vi "KB-CalArrayPointXY.vi"(6 "子数组":dbl[][](array[numeric]), 8 "error in (no error)":errorcluster caption="错误输入（无错误）", 9 "Point":cluster{"X":dbl, "Y":dbl, "Z":dbl}[](array[cluster]), 11 "Image In":T1(plugin-control)) -> (0 "error out":errorcluster caption="错误输出", 1 "Z1-Z2":dbl, 2 "H":string, 3 "Image Out":T1(plugin-control), 4 "对角面最高点":cluster{"X":dbl, "Y":dbl, "Z":dbl})   [LabVIEW 2015]
uses:
  <vilib>/Math Plots/3D Math Plots/3D Surface/3D Surface XCtrl/3D Surface.xctl
  <vilib>/Math Plots/3D Math Plots/3D Surface/3D Surface Datatype/Public/Plot Helper (Matrix).vi
  <vilib>/Math Plots/3D Math Plots/3D Surface/3D Surface Datatype/3D Surface Datatype.lvclass
panel:
  out "子数组 3":dbl[][](array[numeric])
  out "3D Surface 3":refnum<class "3D Plot Datatype.lvclass">[](xcontrol) caption="三维曲面"
  out "最大值":dbl
  out "最大索引":i32[](array[numeric])
  out "3D Surface 2":refnum<class "3D Plot Datatype.lvclass">[](xcontrol) caption="三维曲面"
  out "3D Surface":refnum<class "3D Plot Datatype.lvclass">[](xcontrol) caption="三维曲面"
  out "元素 3":dbl
  out "子数组 2":dbl[][](array[numeric])
  out "x与y？ 4":bool
  out "x与y？ 3":bool
  out "x与y？ 2":bool
  out "x与y？":bool
  out "数字":u32
  out "2R":i32
  out "大小":i32[](array[numeric])
  out "最高点":cluster{"X":dbl, "Y":dbl, "Z":dbl}
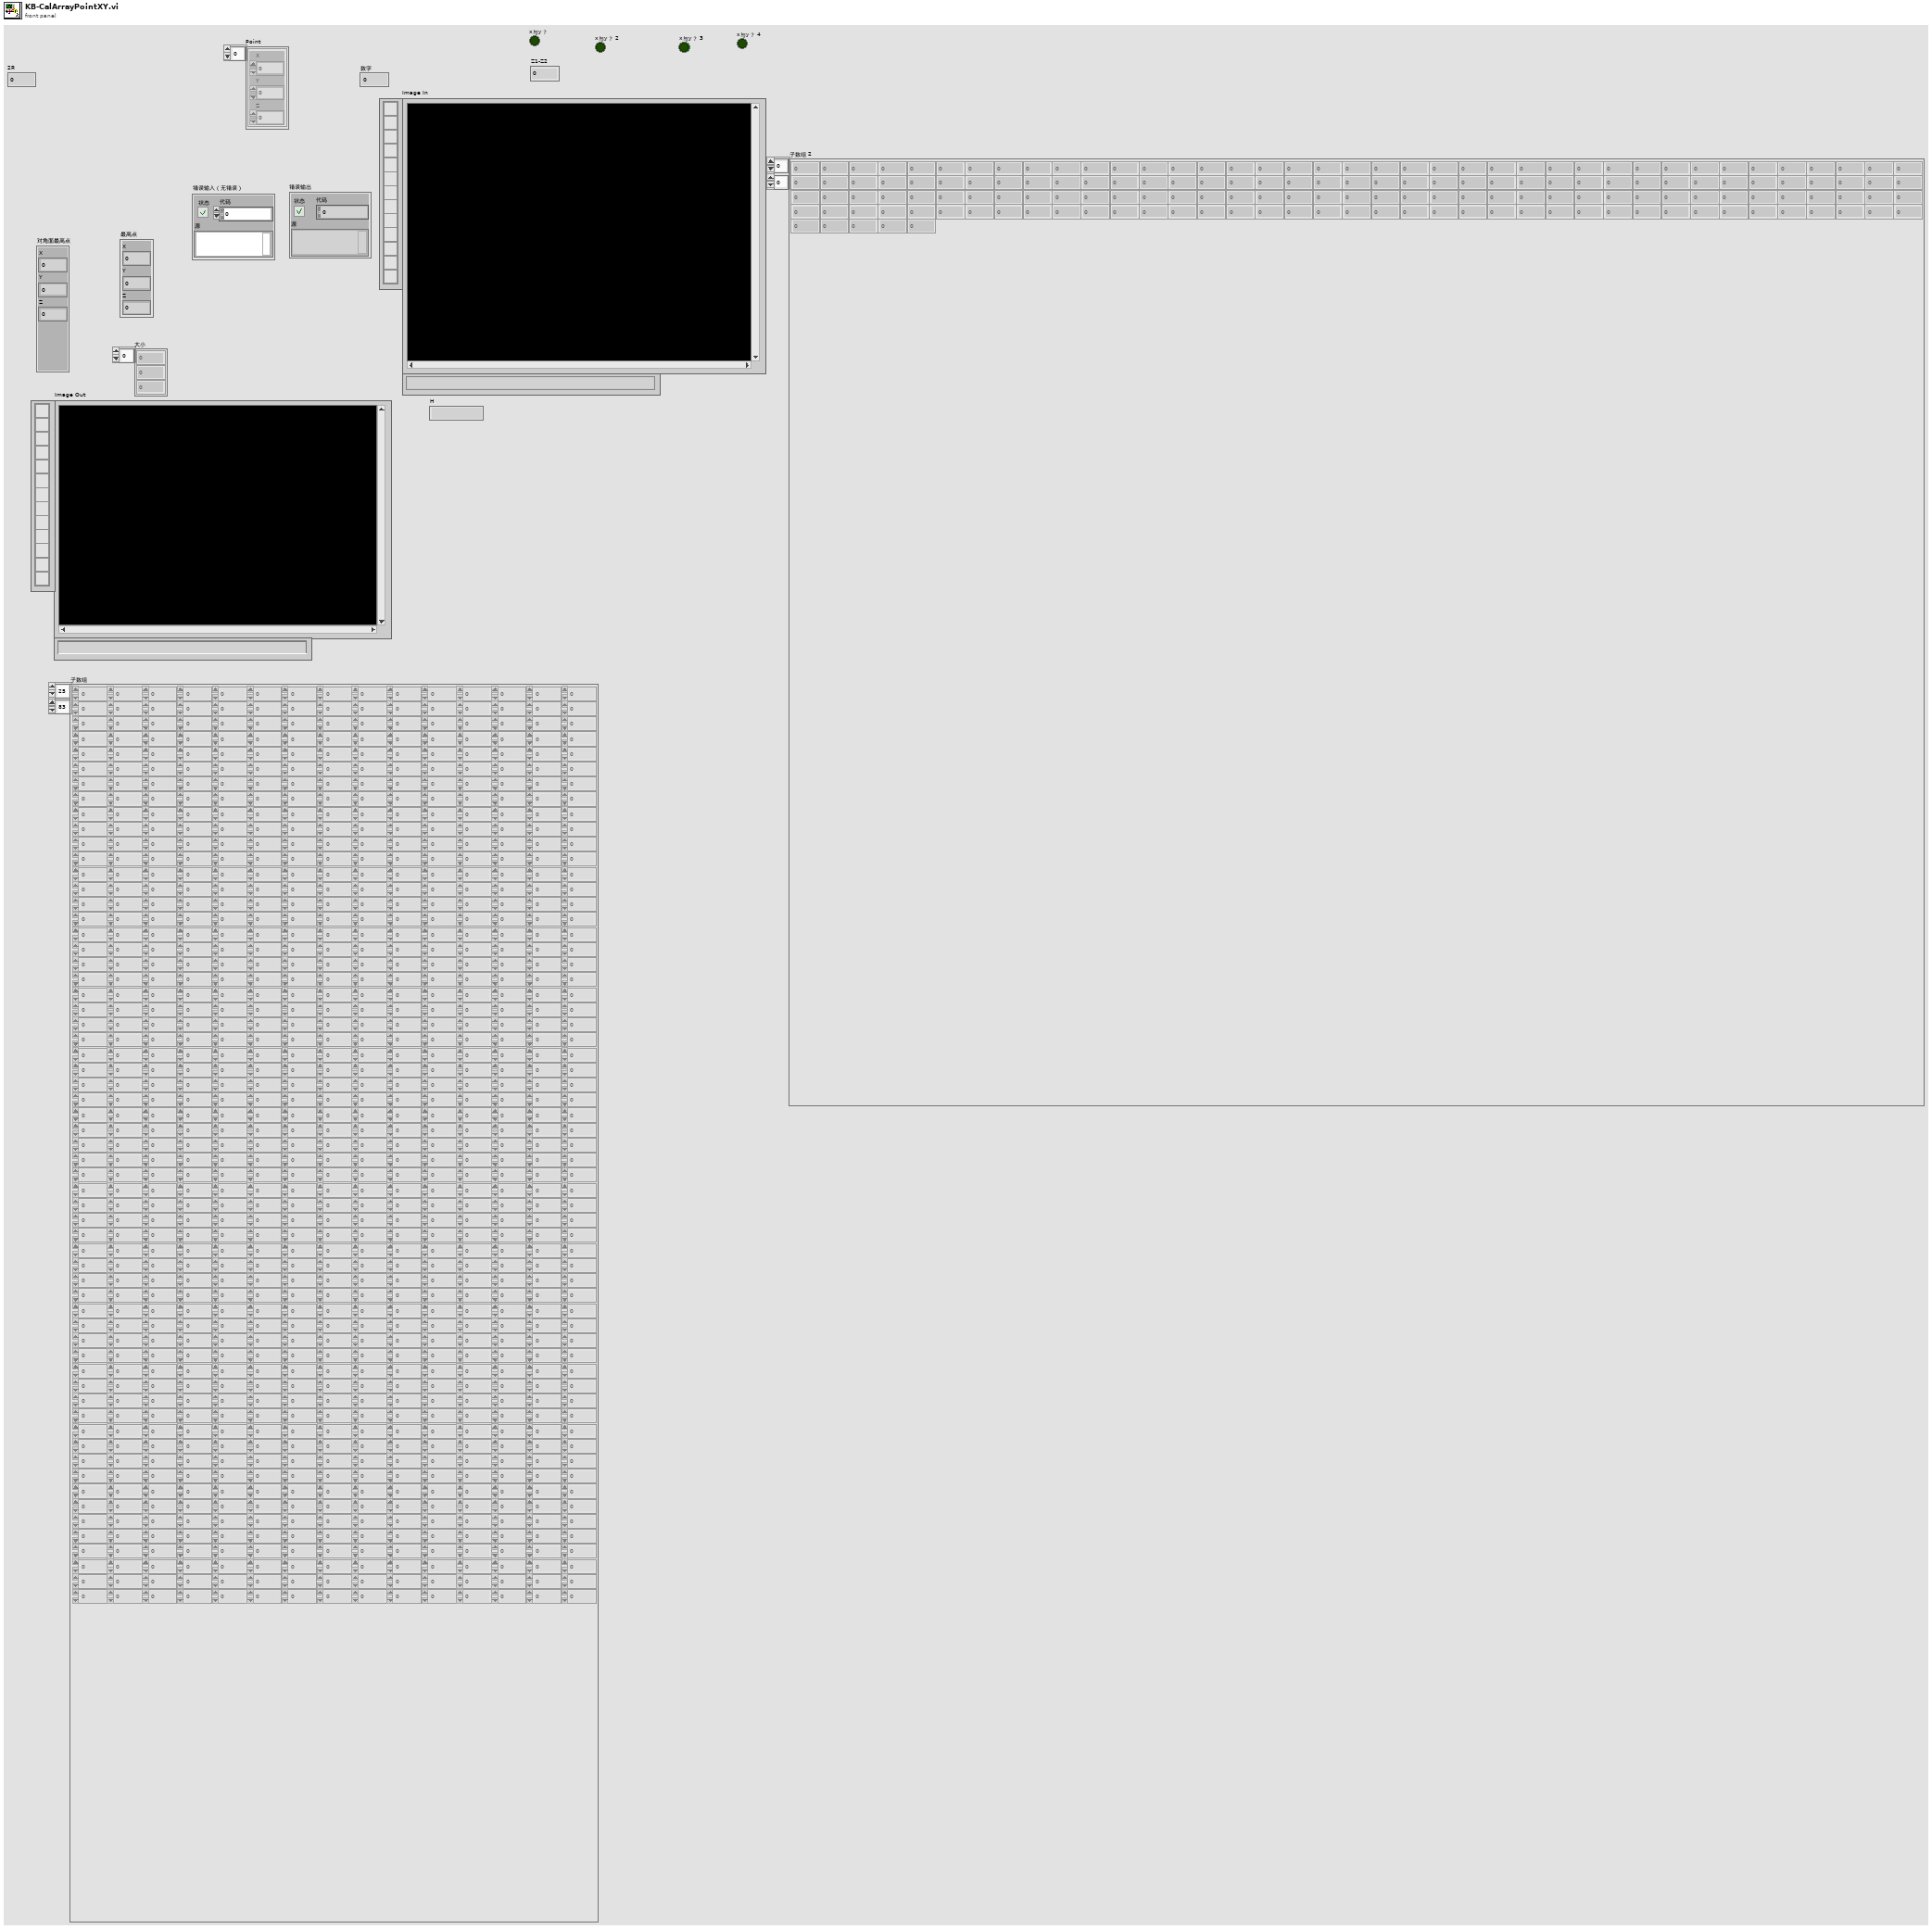
[diagram p1: front panel]
types:
  T1 = typedef "IMAQ Image.ctl" = refnum<image>
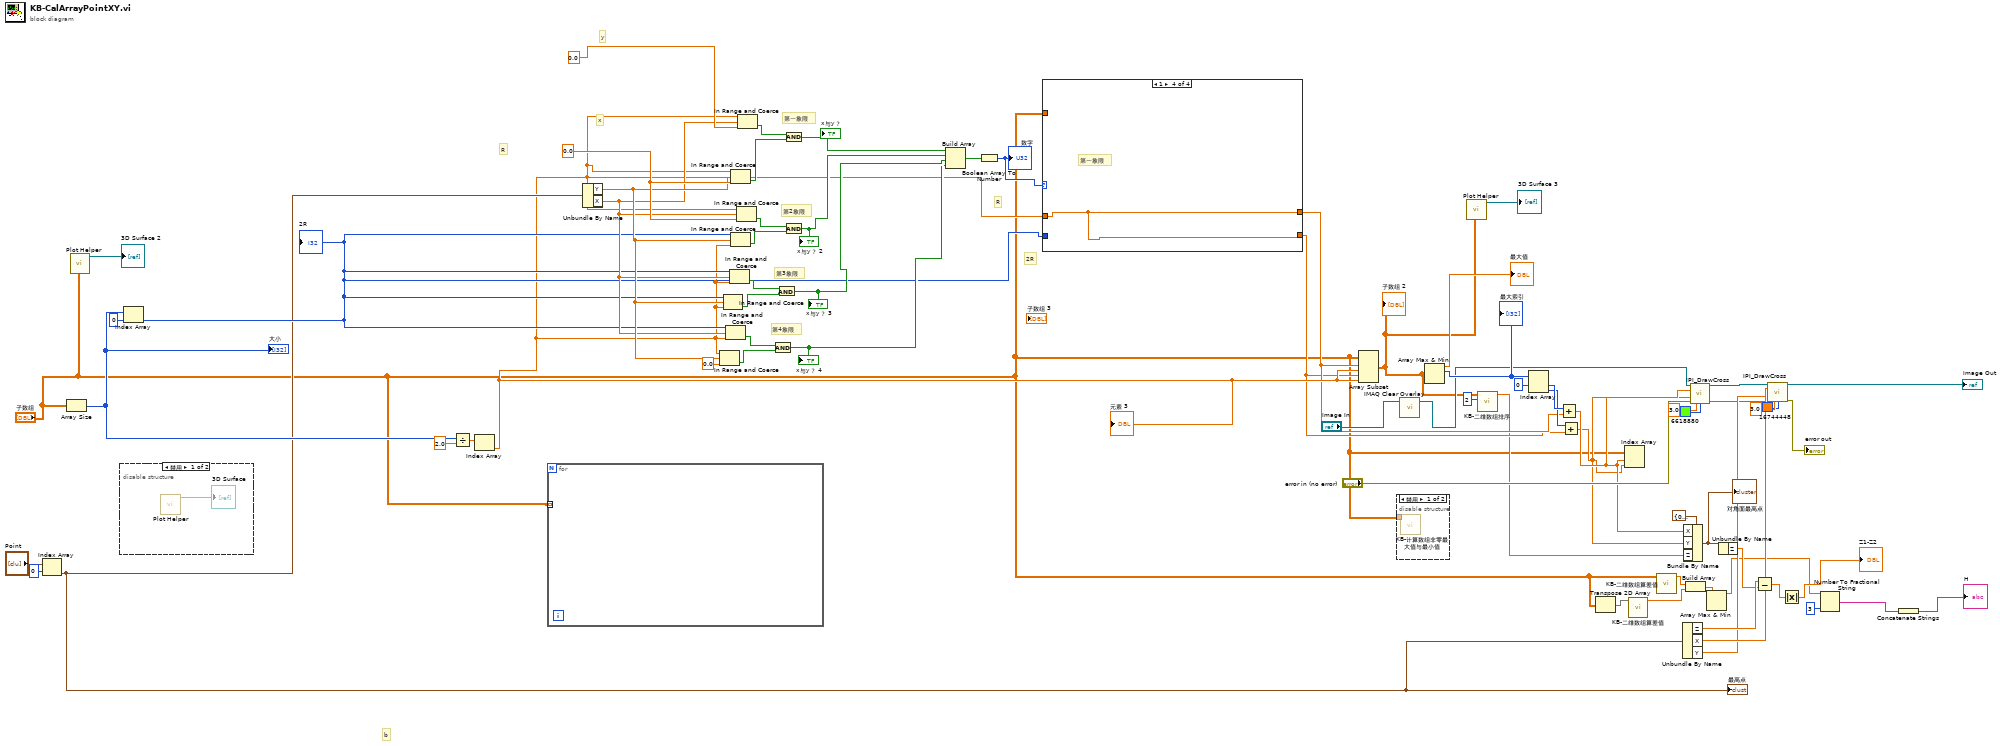
[diagram p0: block diagram]
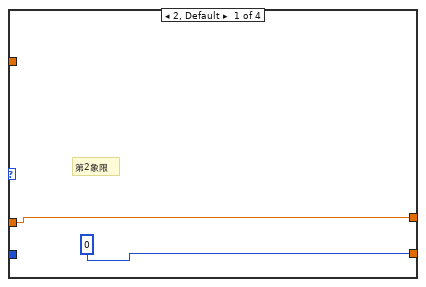
[diagram p4: hidden frame]
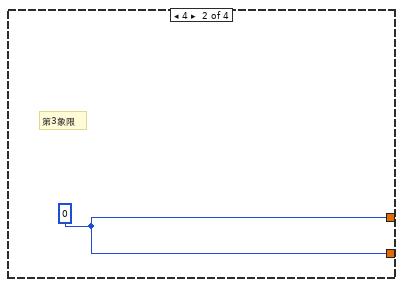
[diagram p5: hidden frame]
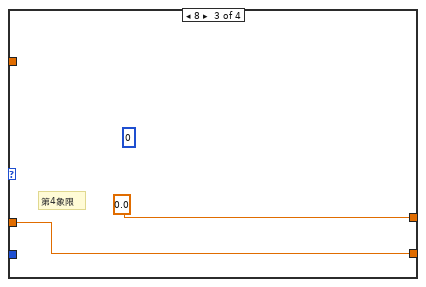
[diagram p6: hidden frame]
diagram:
  w54 = 0.0 ("元素")
  # "2R"
  # "R"
  # "第4象限"
  # "第3象限"
  # "R"
  # "第2象限"
  # "第一象限"
  # "y"
  # "x"
  # "b"
  n1 = Index Array(array="Point", index=0 ("索引")) -> (element=w30:cluster{"X":dbl, "Y":dbl, "Z":dbl})
  "最高点" <- w30
  n2 = Array Size(array="子数组") -> (size(s)=w58:i32[])
  "大小" <- w58
  n3 = call-poly <vilib>:"Plot Helper.vi"("z matrix"="子数组") -> ("3D Plot lvclass Array out"=→"3D Surface 2":refnum<class "3D Plot Datatype.lvclass">[])  [unwired: 5 in, 5 out]
  n4 = disable-structure shown="禁用" {
    frame Disabled {
      n5 = call-poly <vilib>:"Plot Helper.vi"() -> ("3D Plot lvclass Array out"=→"3D Surface":refnum<class "3D Plot Datatype.lvclass">[])  [unwired: 6 in, 5 out]
    }
    frame Enabled {
    }
  }
  n6 = Index Array(array=w58, index=0 ("索引")) -> (element=w42:i32)
  "2R" <- w42
  n7 = Divide(x=w58, y=2.0) -> (x/y=w64:dbl[])
  n8 = Index Array(array=w64) -> (element=w21:dbl)  [unwired: 1 in]
  "元素 3" <- w21
  n9 = for {
    tunnel: "子数组" -> [_] mode=indexing
  }
  n10 = Unbundle By Name(w30) -> ("Y"=w51:dbl, "X"=w49:dbl)
  n11 = In Range and Coerce(upper limit=w21, x=w51, lower limit=0.0 ("下限")) -> (In Range?=w53:bool)  [unwired: 1 out]
  n12 = In Range and Coerce(upper limit=w42, x=w51, lower limit=w21) -> (In Range?=w55:bool)  [unwired: 1 out]
  n13 = In Range and Coerce(upper limit=w42, x=w49, lower limit=w21) -> (In Range?=w52:bool)  [unwired: 1 out]
  n14 = In Range and Coerce(upper limit=w42, x=w49, lower limit=w21) -> (In Range?=w56:bool)  [unwired: 1 out]
  n15 = In Range and Coerce(upper limit=w42, x=w51, lower limit=w21) -> (In Range?=w60:bool)  [unwired: 1 out]
  n16 = In Range and Coerce(upper limit=w21, x=w51, lower limit=w54) -> (In Range?=w61:bool)  [unwired: 1 out]
  n17 = In Range and Coerce(upper limit=w21, x=w49, lower limit=w54) -> (In Range?=w59:bool)  [unwired: 1 out]
  n18 = In Range and Coerce(upper limit=w21, x=w49, lower limit=0.0 ("元素")) -> (In Range?=w62:bool)  [unwired: 1 out]
  n19 = And(x=w52, y=w53) -> (x .and. y?=w45:bool)
  "x与y？ 4" <- w45
  n20 = And(x=w56, y=w55) -> (x .and. y?=w46:bool)
  "x与y？ 3" <- w46
  n21 = And(x=w62, y=w61) -> (x .and. y?=w48:bool)
  "x与y？" <- w48
  n22 = And(x=w59, y=w60) -> (x .and. y?=w47:bool)
  "x与y？ 2" <- w47
  n23 = Build Array(w48, w47, w46, w45) -> (w44:bool[])
  n24 = Boolean Array To Number(Boolean array=w44) -> (number=w43:u32)
  "数字" <- w43
  n25 = case shown="1" w43 {
    tunnel: [w72 w74 0.0 w77] -> w15
    tunnel: [0 w74 w75 w77] -> w14
    tunnel: w21 -> [w72 _ w75 w77]
    tunnel: w42 -> [_ _ _ _]
    tunnel: "子数组" -> [_ _ _ _]
    frame 2, Default {
      # "第2象限"
    }
    frame 4 {
      w74 = 0
      # "第3象限"
    }
    frame 8 {
      (unwired) 0 ("行")
      # "第4象限"
    }
    frame 1 {
      # "第一象限"
    }
  }
  n26 = Array Subset(array="子数组", index (row)=w15, length (row)=w21, index (col)=w14, length (col)=w21) -> (w9:dbl[][])
  "子数组 2" <- w9
  n27 = disable-structure shown="禁用" {
    disable-tunnel: "子数组" -> [w78 _]
    frame Disabled {
      n28 = call "KB-计算数组非零最大值与最小值.vi"("原始数据"=w78) -> ()  [unwired: 9 in, 2 out]
    }
    frame Enabled {
    }
  }
  n29 = call "IMAQ Clear Overlay"("Image"="Image In") -> ("Image Out"=w12:T1)  [unwired: 9 in, 1 out]
  n30 = Array Max & Min(array=w9) -> (max value=→"最大值":dbl, max index (indices)=w41:i32[])  [unwired: 2 out]
  "最大索引" <- w41
  n31 = call-poly <vilib>:"Plot Helper.vi"("z matrix"=w9) -> ("3D Plot lvclass Array out"=→"3D Surface 3":refnum<class "3D Plot Datatype.lvclass">[])  [unwired: 5 in, 5 out]
  n32 = call "KB-二维数组排序.vi"("平均个数"=2, "二维数组"=w9) -> ("平均最高值"=w7:dbl)  [unwired: 9 in]
  n33 = Index Array(array=w41, index #1=0 ("索引")) -> (element #1=w20:i32, element #2=w19:i32)  [unwired: 1 in]
  n34 = Add(x=w20, y=w15) -> (x+y=w11:dbl)
  n35 = Add(x=w19, y=w14) -> (x+y=w10:dbl)
  n36 = Transpose 2D Array(2D array="子数组") -> (transposed array=w1:dbl[][])
  n37 = Index Array(array="子数组", index (row)=w11, index (col)=w10) -> ()  [unwired: 1 out]
  n38 = call "KB-二维数组算差值.vi"("子数组"=w1) -> ("差值"=w5:dbl)  [unwired: 10 in]
  n39 = call "KB-二维数组算差值.vi"("子数组"="子数组") -> ("差值"=w6:dbl)  [unwired: 10 in]
  n40 = Unbundle By Name(w30) -> ("Z"=w67:dbl, "X"=w29:dbl, "Y"=w28:dbl)
  n41 = Bundle By Name(cluster=cluster{"X":dbl, "Y":dbl, "Z":dbl} {"X"=0.0, "Y"=0.0, "Z"=0.0}, "X"=w11, "Y"=w10, "Z"=w7) -> (w17:cluster{"X":dbl, "Y":dbl, "Z":dbl})
  "对角面最高点" <- w17
  n42 = Build Array(w6, w5) -> (w4:dbl[])
  n43 = call "IPI_DrawCross.vi"("Image In"=w12, "X"=w11, "Y"=w10, "error in (no error)"="error in (no error)", "Radius"=3.0, "颜色盒"=u32 6618880) -> ("Image Out"=w32:T1, "error out"=w27:errorcluster)  [unwired: 8 in]
  n44 = Array Max & Min(array=w4) -> (max value=w3:dbl)  [unwired: 3 out]
  n45 = Unbundle By Name(w17) -> ("Z"=w66:dbl)
  n46 = Subtract(x=w67, y=w66) -> (x-y=w38:dbl)
  n47 = call "IPI_DrawCross.vi"("Image In"=w32, "X"=w29, "Y"=w28, "error in (no error)"=w27, "Radius"=3.0, "颜色盒"=u32 16744448) -> ("Image Out"=→"Image Out":T1, "error out"=→"error out":errorcluster)  [unwired: 8 in]
  n48 = Absolute Value(x=w38) -> (abs(x)=→"Z1-Z2":dbl)
  n49 = Number To Fractional String(number=w3, precision (6)=i16 3 ("精度(6)")) -> (F-format string=w35:string)  [unwired: 2 in]
  n50 = Concatenate Strings(w35) -> (→"H":string)
